vi "count rate.vi"() -> ()   [LabVIEW 2014]
uses:
  <vilib>/Platform/TimedLoop/XDataNode/timing_clust.ctl
  <vilib>/Platform/TimedLoop/XDataNode/nitl_modes.ctl
  <vilib>/Platform/TimedLoop/XDataNode/wakeup.ctl
  <vilib>/Waveform/WDTFileIO.llb/ Write Waveform to File.vi
  <vilib>/platform/TimedLoop/XDataNode/XDataNode.xnode
  <vilib>/Platform/TimedLoop/XDataNode/XDNodeRunTimeDep.lvlib
panel:
  in  "file path (use dialog)":path=path "C:/Users/davidb52/Desktop/week8/decay"
  in  "Period (s)":dbl=1.0
  in  "Aquisition time":dbl=300.0
  out "Waveform Graph":waveform(i32)(graph)={"t0"=timestamp(0 s since 1904-01-01), "dt"=1.0, "Y"=[0, 20, 26, 13, 18, 29, 19, 33, 24, 22, 23, 28, 31, 24, 26, 18, 31, 28, 30, 20, 25, 30, 33, 38, 29, 28, 39, 30, 29, 33, 38, 28, 37, 30, 43, 28, 40, 30, 33, 31, 34, 49, 31, 41, 39, 29, 23, 31, 28, 30, 33, 39, 43, 37, 21, 30, 29, 30, 34, 21, 37, 35, 30, 17, 24, 32, 29, 32, 24, 26, 30, 20, 26, 35, 26, 20, 27, 29, 24, 22, 20, 22, 24, 13, 26, 24, 32, 23, 24, 28, 16, 27, 27, 30, 25, 28, 26, 22, 22, 19, 10, 19, 23, 23, 28, 20, 17, 15, 13, 23, 18, 28, 24, 13, 16, 26, 21, 26, 13, 23, 8, 11, 18, 13, 14, 12, 13, 15, 23, 12, 14, 16, 20, 20, 13, 12, 18, 15, 14, 19, 20, 21, 19, 13, 12, 9, 9, 18, 14, 12, 12, 14, 10, 18, 15, 12, 17, 15, 18, 12, 6, 12, 10, 16, 9, 18, 12, 9, 9, 9, 14, 15, 11, 11, 11, 9, 5, 10, 15, 17, 8, 15, 8, 6, 10, 5, 8, 8, 9, 8, 10, 10, 13, 10, 15, 10, 9, 4, 14, 9, 11, 14, 12, 7, 11, 12, 15, 16, 7, 12, 15, 10, 8, 6, 15, 6, 7, 9, 12, 6, 12, 9, 8, 7, 10, 4, 10, 7, 14, 7, 7, 6, 10, 11, 6, 9, 12, 5, 12, 12, 6, 6, 3, 4, 4, 7, 5, 3, 8, 8, 8, 10, 9, 11, 7, 9, 2, 9, 8, 10, 9, 7, 4, 10, 5, 5, 7, 7, 2, 6, 8, 8, 8, 7, 5, 5, 2, 10, 11, 5, 3, 6, 5, 7, 10, 9, 5, 10, 7, 5, 1, 5, 8, 2, 5, 4, 4, 7, 10, 9, 2]}
  in  "stop":bool
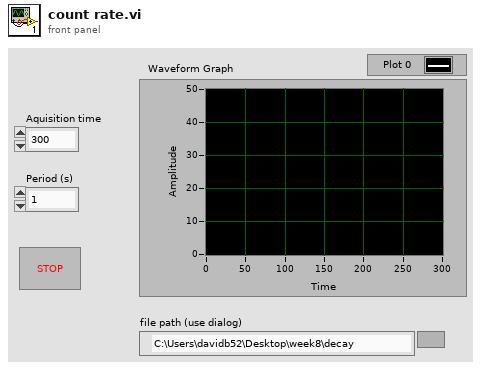
[diagram p1: front panel]
types:
  T1 = typedef "XDNodeRunTimeDep.lvlib/timing_clust.ctl" = cluster{"Expected End [f-1]":u64, "Actual End [f-1]":u64, "Finished Late? [f-1]":bool, "Expected End [i-1]":u64, "Actual End [i-1]":u64, "Finished Late? [i-1]":bool, "Expected Start [i]":u64, "Actual Start [i]":u64, "Expected Start [f]":u64, "Actual Start [f]":u64, "Source Name":string, "Structure Name":string, "Period":i64, "Deadline":i64, "Offset":i64, "Start":i64, "Priority":i32, "Timeout":i32, "Mode":T2, "Wakeup Reason":T3, "Error":errorcluster, "Source Type":string, "Secondary Source Type":string, "Global End Time":u64, "Global Start Time":u64, "Frame Duration":u64, "Iteration Duration":u64, "Assigned CPU":i32, "I/O Scan Engine Mode":u32}
  T2 = typedef "XDNodeRunTimeDep.lvlib/nitl_modes.ctl" = enum32{"No Change", "Process missed periods, maintain original phase", "Discard missed periods, maintain original phase", "Process missed periods, ignore original phase", "Discard missed periods, ignore original phase"}
  T3 = typedef "XDNodeRunTimeDep.lvlib/wakeup.ctl" = enum32{"Normal", "Aborted", "Asynchronous wakeup", "Timing source error", "Timed loop error", "Timeout"}
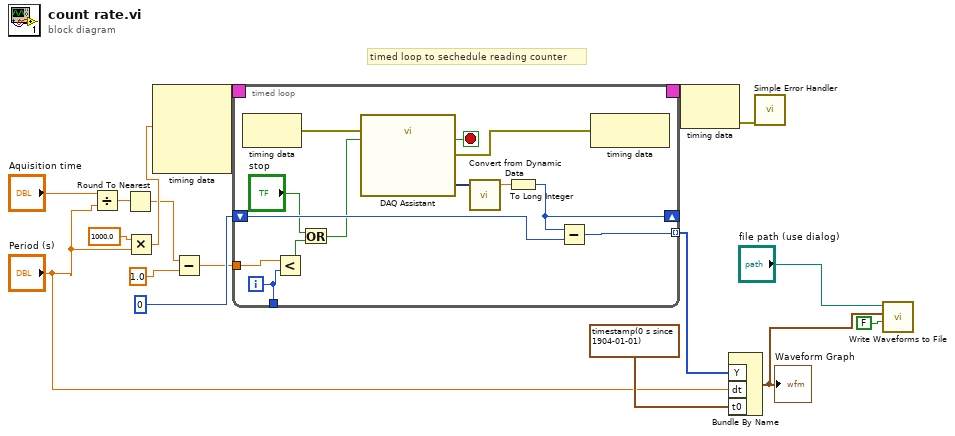
[diagram p0: block diagram]
diagram:
  # "timed loop to sechedule reading counter"
  n1 = Divide(x="Aquisition time", y="Period (s)") -> (x/y=w6:dbl)
  n2 = Round To Nearest(number=w6) -> (nearest integer value=w10:dbl)
  n3 = Multiply(x=1000.0, y="Period (s)") -> (x*y=w13:dbl)
  n4 = node-c288(w13) -> (w17:T1)  [unwired: 3 in]
  n5 = Subtract(x=w10, y=1.0) -> (x-y=w9:dbl)
  n6 = timed-loop {
    timing: w17 -> [_]
    timing-out: [_] -> w16
    shift-right: [w27] -> _
    shift-left: 0 -> [w29]
    tunnel: [w23] -> w7 mode=indexing
    tunnel: w9 -> [w22]
    tunnel: [w18] -> _
    i -> [w18]
    stop <- w28 stop-if-true
    n7 = node-c288() -> (w24:errorcluster)  [unwired: 1 in]
    n8 = Less?(x=w22, y=w18) -> (x < y?=w21:bool)
    n9 = Or(x="stop", y=w21) -> (x .or. y?=w19:bool)
    n10 = call "DAQ Assistant"("error in"=w24, "stop (F)"=w19) -> ("data"=w30:dynamicdata, "stopped"=w28:bool, "error out"=w25:errorcluster)  [unwired: 14 in, 1 out]
    n11 = call "Convert from Dynamic Data"("Dynamic Data Type"=w30) -> ("Scalar"=w26:dbl)  [unwired: 3 in]
    n12 = To Long Integer(number=w26) -> (32bit integer=w27:i32)
    n13 = Subtract(x=w27, y=w29) -> (x-y=w23:i32)
    n14 = node-c288(w25) -> ()  [unwired: 1 out]
  }
  n15 = node-c288(w16) -> (w14:errorcluster)
  n16 = Bundle By Name("Y"=w7, "dt"="Period (s)", "t0"=timestamp(0 s since 1904-01-01)) -> (w1:waveform(i32))  [unwired: 1 in]
  "Waveform Graph" <- w1
  n17 = call <vilib>:"Simple Error Handler.vi"("error in (no error)"=w14) -> ()  [unwired: 4 in, 5 out]
  n18 = call-poly <vilib>:"Write Waveforms to File.vi"("append to file? (new file:F)"=FALSE, "waveform"=w1, "file path (dialog if empty)"="file path (use dialog)") -> ()  [unwired: 7 in, 2 out]
